vi "Wait for Parameter.vi"(6 "Auto-resolve Error (T)":bool=TRUE, 7 "Param Type (Default)":refnum<class>, 8 "error in (no error)":errorcluster, 9 "Timeout mS (-1)":i32=-1, 11 "Promise in":refnum<class "Promise.lvclass">) -> (0 "error out":errorcluster, 2 "Parameter":refnum<class>, 3 "Promise out":refnum<class "Promise.lvclass">)   [LabVIEW 2020, in "Promises.lvlib" / "Promise.lvclass"]
doc: "Waits for the input parameter for the task to be received, optionally with a timeout. If an error is provided, such as from Promise chaining or the wait times out, then the Promise will automatically be resolved with an error and the calling task does not need to resolve the task itself."
uses:
  Promise.lvclass
  Promise.lvclass/Promise.ctl
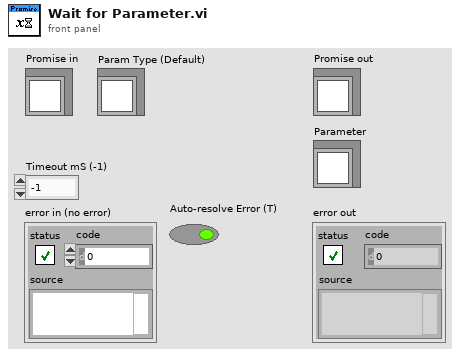
[diagram p1: front panel]
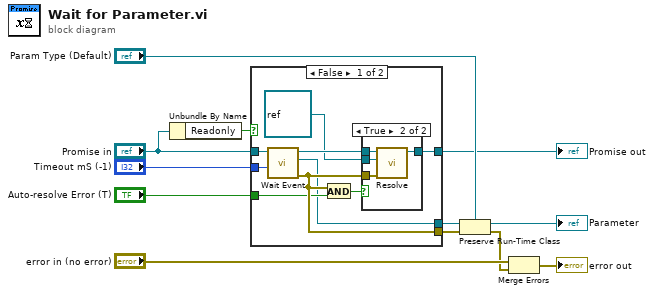
[diagram p0: block diagram]
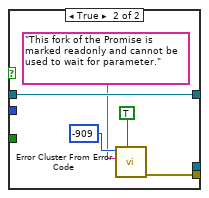
[diagram p3: hidden frame]
diagram:
  n1 = Unbundle By Name("Promise in") -> ("Readonly"=w1:bool)
  n2 = case shown="False" w1 {
    tunnel: "Promise in" -> [w20 w31]
    tunnel: "Timeout mS (-1)" -> [w19 _]
    tunnel: [w17 w31] -> w8
    tunnel: "Auto-resolve Error (T)" -> [w15 _]
    tunnel: [w21 w30] -> w4
    tunnel: [w14 _] -> w3
    frame False {
      n3 = call "Wait Event.vi"("Timeout mS (-1)"=w19, "Promise in"=w20) -> ("error out"=w21:errorcluster, "Value"=w14:refnum<class>, "Promise out"=w18:refnum<class "Promise.lvclass">)  [unwired: 7 in]
      n4 = And(x=w21, y=w15) -> (x .and. y?=w16:bool)
      n5 = case shown="True" w16 {
        tunnel: w18 -> [w22 w26]
        tunnel: refnum<class> refnum ("LabVIEW Object") -> [_ w25]
        tunnel: [w22 w24] -> w17
        tunnel: w21 -> [_ w23]
        frame False {
        }
        frame True {
          n6 = call "Resolve.vi"("error in (no error)"=w23, "Result (None)"=w25, "Promise in"=w26) -> ("Promise in"=w24:refnum<class "Promise.lvclass">)  [unwired: 7 in, 1 out]
        }
      }
    }
    frame True {
      n7 = call <vilib>:"Error Cluster From Error Code.vi"("show call chain? (False)"=TRUE, "error message (\"\")"="This fork of the Promise is marked readonly and cannot be used to wait for parameter.", "error code (0)"=-909) -> ("error out"=w30:errorcluster)  [unwired: 6 in]
    }
  }
  "Promise out" <- w8
  n8 = Preserve Run-Time Class(object in=w3, error in=w4, 2:"Param Type (Default)") -> (object out=→"Parameter":refnum<class>, error out=w5:errorcluster)
  n9 = Merge Errors("error in (no error)", w5) -> (→"error out":errorcluster)
